vi "_TEST.vi"(8 "error in (no error)":errorcluster, 9 "height":dbl=2.0, 10 "breadth":dbl=3.0, 11 "length":dbl=4.0) -> (0 "error out":errorcluster, 2 "volumn":dbl, 3 "area":dbl)   [LabVIEW 2020]
uses:
  box.lvlib
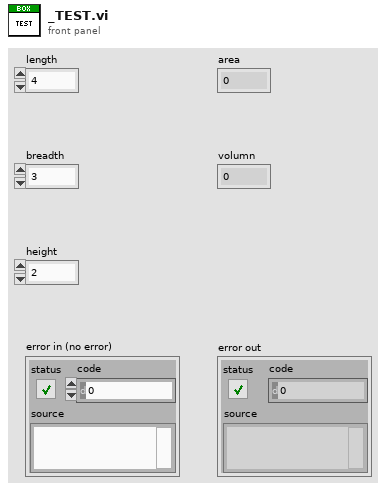
[diagram p1: front panel]
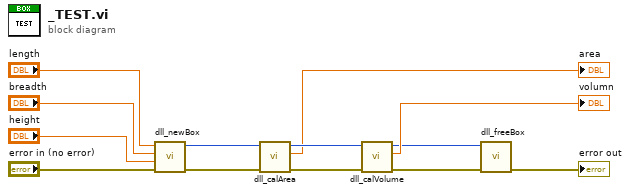
[diagram p0: block diagram]
diagram:
  n1 = call "dll_newBox.vi"("error in (no error)"="error in (no error)", "height"="height", "breadth"="breadth", "length"="length") -> ("error out"=w11:errorcluster, "p_box"=w13:i32)  [unwired: 6 in]
  n2 = call "dll_calArea.vi"("error in (no error)"=w11, "p_box"=w13) -> ("error out"=w10:errorcluster, "area"=→"area":dbl, "p_box"=w12:i32)  [unwired: 7 in]
  n3 = call "dll_calVolume.vi"("error in (no error)"=w10, "p_box"=w12) -> ("error out"=w2:errorcluster, "volumn"=→"volumn":dbl, "p_box"=w3:i32)  [unwired: 7 in]
  n4 = call "dll_freeBox.vi"("error in (no error)"=w2, "p_box"=w3) -> ("error out"=→"error out":errorcluster)  [unwired: 9 in]
